vi "Data_Array_Read.vi"(8 "error in (no error)":errorcluster, 11 "Data_Array in":refnum<class "Data_Array.lvclass">) -> (0 "error out":errorcluster, 2 "Data_params":cluster{"Data":dbl[], "Index":i32, "Buffer":i32}, 3 "Data_Array out":refnum<class "Data_Array.lvclass">)   [LabVIEW 2021, in "Data_Array.lvclass"]
uses:
  Data_Array.lvclass
  Data_Array.lvclass/Data_Array.ctl
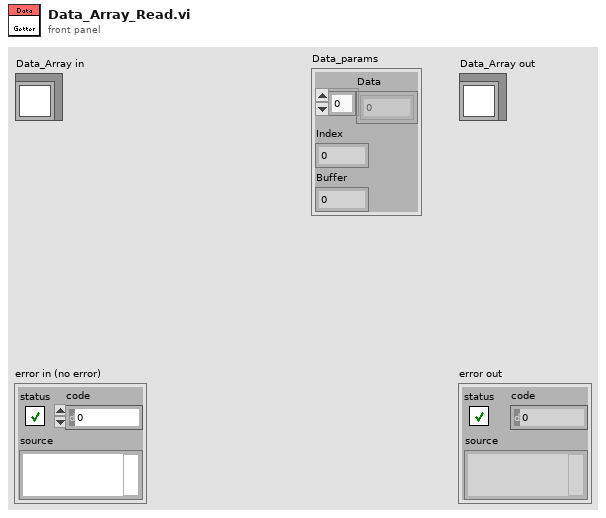
[diagram p1: front panel]
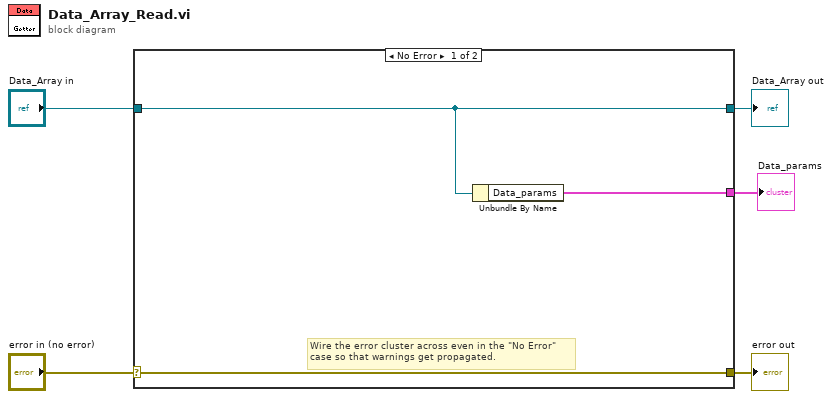
[diagram p0: block diagram]
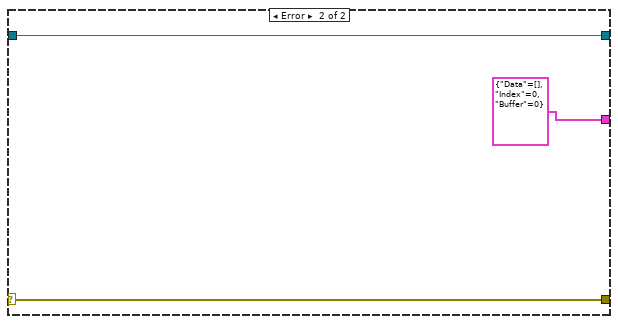
[diagram p2: hidden frame]
diagram:
  n1 = case shown="No Error" "error in (no error)" {
    selector: "error in (no error)" -> [w8 w11]
    tunnel: [w8 w11] -> w4
    tunnel: [w7 w10] -> w2
    tunnel: "Data_Array in" -> [w7 w10]
    tunnel: [w6 cluster{"Data":dbl[], "Index":i32, "Buffer":i32} {"Data"=[], "Index"=0, "Buffer"=0} ("Data_params")] -> w1
    frame No Error {
      # "Wire the error cluster across even in the \"No Error\"\ncase so that warnings get propagated."
      n2 = Unbundle By Name(w7) -> ("Data_params"=w6:cluster{"Data":dbl[], "Index":i32, "Buffer":i32})
    }
    frame Error {
    }
  }
  "error out" <- w4
  "Data_Array out" <- w2
  "Data_params" <- w1
